vi "Insert Instrument Class by Name.vi"(8 "error in (no error)":errorcluster, 9 "Type":T1, 10 "Instrument in":refnum<class "Instrument.lvclass">, 11 "Control Experiment in":refnum<class "Control Experiment.lvclass">) -> (0 "error out":errorcluster, 1 "Found?":bool, 2 "Instrument out":refnum<class "Instrument.lvclass">, 3 "Control Experiment out":refnum<class "Control Experiment.lvclass">)   [LabVIEW 2019, in "Control Experiment.lvclass"]
uses:
  Control Experiment.lvclass
  Typedefs/Instrument Types--combo.ctl
  <userlib>/LevyLab/Instrument Framework/SMOs/Instrument/Instrument.lvclass
  Typedefs/Instruments--cluster.ctl
  <userlib>/LevyLab/Krohn Hite 7008/Instrument.KH7008.lvclass
  <userlib>/LevyLab/Lockin-Multichannel/Instrument.Lockin/Instrument.Lockin.lvclass
  <userlib>/LevyLab/Instrument Framework/Instrument Types/Cryostat/Instrument.Cryostat.lvclass
  <userlib>/LevyLab/Instrument Framework/Instrument Types/CBridge/Instrument.CBridge.lvclass
  <userlib>/LevyLab/Instrument Framework/Instrument Types/Delay Line/Instrument.DelayLine.lvclass
  <userlib>/LevyLab/Instrument Framework/Instrument Types/Strain/Instrument.Strain.lvclass
  <userlib>/LevyLab/Instrument Framework/Instrument Types/VNA/Instrument.VNA.lvclass
  <userlib>/LevyLab/Instrument Framework/Instrument Types/VSource/Instrument.VSource.lvclass
  Control Experiment.lvclass/Control Experiment.ctl
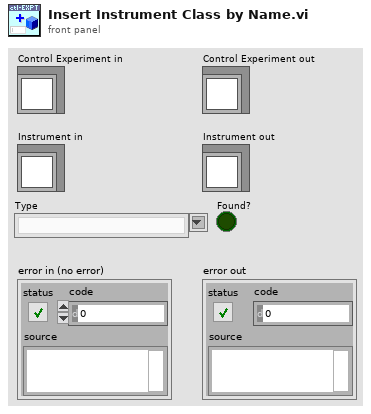
[diagram p1: front panel]
types:
  T1 = typedef "Control Experiment.lvclass/Instrument Types--combo.ctl" = string
  T2 = typedef "Control Experiment.lvclass/Instruments--cluster.ctl" = cluster{"KH7008":refnum<class "Instrument.KH7008.lvclass">[], "Lockin":refnum<class "Instrument.Lockin.lvclass">, "Temperature":refnum<class "Instrument.Cryostat.lvclass">, "Magnet":refnum<class "Instrument.Cryostat.lvclass">, "Rotator":refnum<class "Instrument.Cryostat.lvclass">, "Level":refnum<class "Instrument.Cryostat.lvclass">, "Capacitance Bridge":refnum<class "Instrument.CBridge.lvclass">, "Delay Line":refnum<class "Instrument.DelayLine.lvclass">, "Strain Cell":refnum<class "Instrument.Strain.lvclass">, "VNA":refnum<class "Instrument.VNA.lvclass">, "Voltage Source":refnum<class "Instrument.VSource.lvclass">}
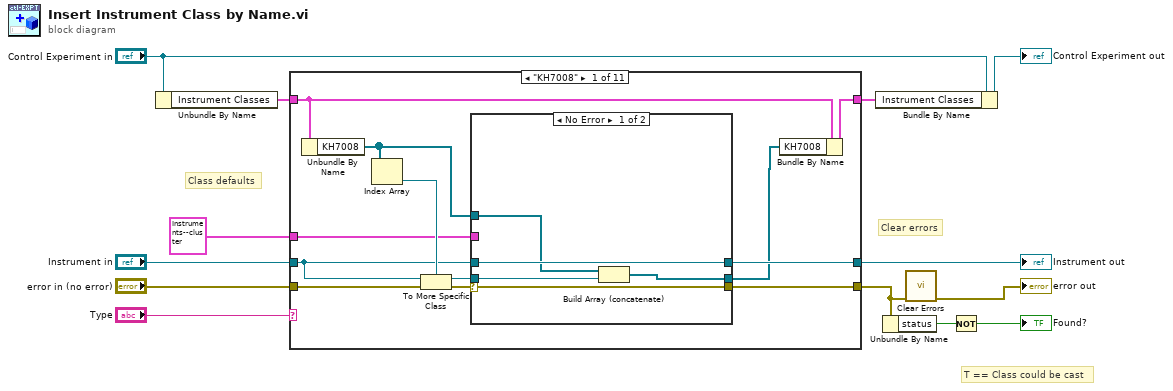
[diagram p0: block diagram]
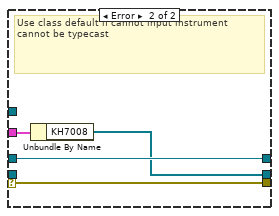
[diagram p2: hidden frame]
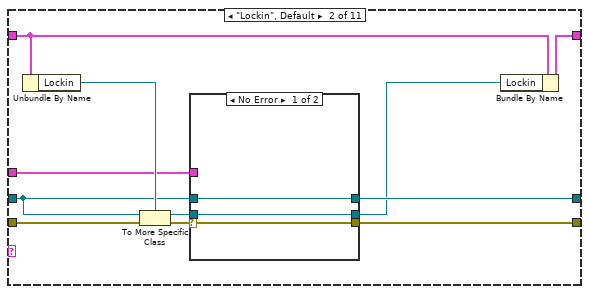
[diagram p3: hidden frame]
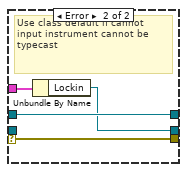
[diagram p4: hidden frame]
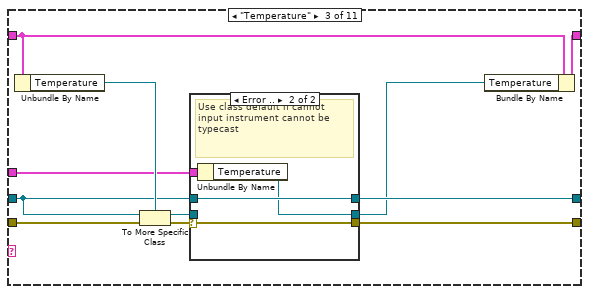
[diagram p5: hidden frame]
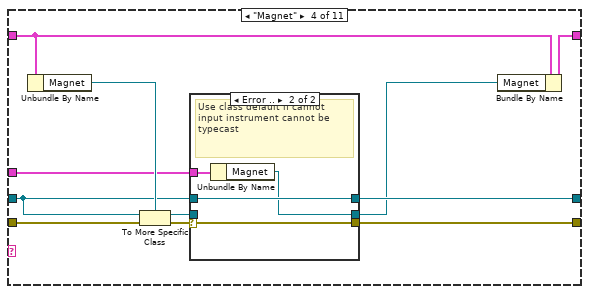
[diagram p7: hidden frame]
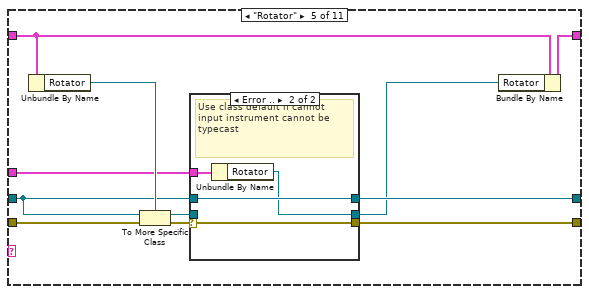
[diagram p9: hidden frame]
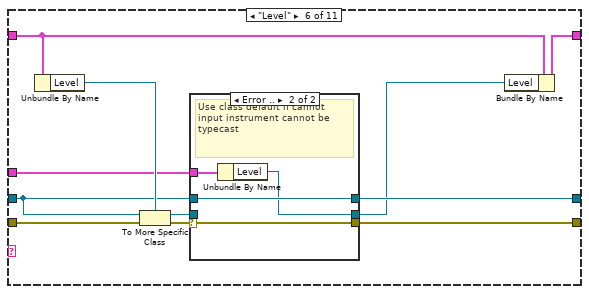
[diagram p11: hidden frame]
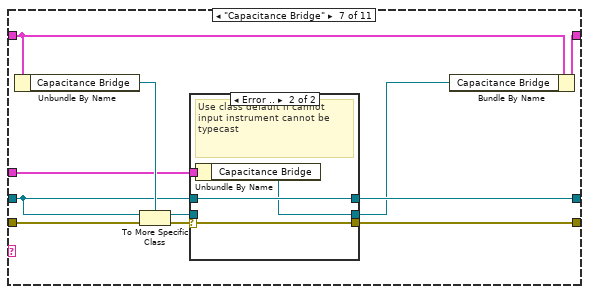
[diagram p13: hidden frame]
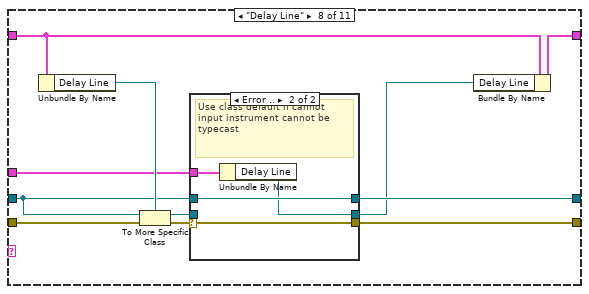
[diagram p15: hidden frame]
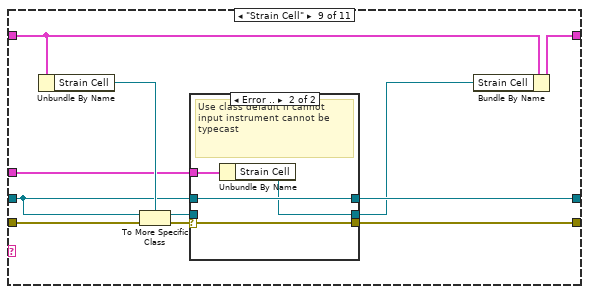
[diagram p17: hidden frame]
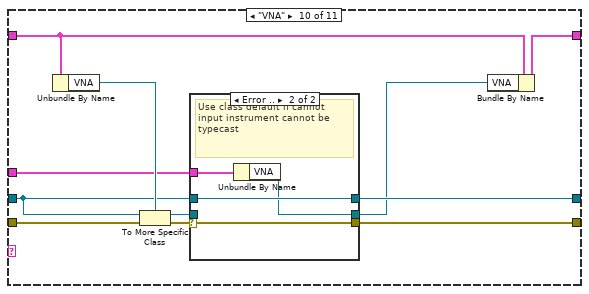
[diagram p19: hidden frame]
diagram:
  # "Class defaults"
  # "T == Class could be cast"
  # "Clear errors"
  n1 = Unbundle By Name("Control Experiment in") -> ("Instrument Classes"=w1:T2)
  n2 = case shown="\"KH7008\"" "Type" {
    tunnel: "Instrument in" -> [w17 w36 w54 w72 w90 w108 w126 w144 w162 w180 w198]
    tunnel: "error in (no error)" -> [w25 w45 w63 w81 w99 w117 w135 w153 w171 w189 w207]
    tunnel: [w16 w38 w56 w74 w92 w110 w128 w146 w164 w182 w200] -> w5
    tunnel: [w19 w39 w57 w75 w93 w111 w129 w147 w165 w183 w201] -> w10
    tunnel: [w23 w43 w61 w79 w97 w115 w133 w151 w169 w187 w205] -> w7
    tunnel: w1 -> [w24 w44 w62 w80 w98 w116 w134 w152 w170 w188 w206]
    tunnel: T2 {"KH7008"=[], "Lockin"=refnum, "Temperature"=refnum, "Magnet"=refnum, "Rotator"=refnum, "Level"=refnum, "Capacitance Bridge"=refnum, "Delay Line"=refnum, "Strain Cell"=refnum, "VNA"=refnum, "Voltage Source"=refnum} ("Instrument Classes") -> [w18 w37 w55 w73 w91 w109 w127 w145 w163 w181 w199]
    frame "KH7008" {
      n3 = Unbundle By Name(w24) -> ("KH7008"=w14:refnum<class "Instrument.KH7008.lvclass">[])
      n4 = Index Array(array=w14) -> (element=w22:refnum<class "Instrument.KH7008.lvclass">)  [unwired: 1 in]
      n5 = To More Specific Class(target class=w22, reference=w17, error in=w25) -> (specific class reference=w20:refnum<class "Instrument.KH7008.lvclass">, error out=w21:errorcluster)
      n6 = case shown="No Error" w21 {
        selector: w21 -> [w29 w33]
        tunnel: w20 -> [w28 _]
        tunnel: [w27 w31] -> w15
        tunnel: [w30 w34] -> w19
        tunnel: w17 -> [w30 w34]
        tunnel: [w29 w33] -> w16
        tunnel: w18 -> [_ w32]
        tunnel: w14 -> [w26 _]
        frame No Error {
          n7 = Build Array (concatenate)(w26, w28) -> (w27:refnum<class "Instrument.KH7008.lvclass">[])
        }
        frame Error {
          # "Use class default if cannot input instrument cannot be typecast"
          n8 = Unbundle By Name(w32) -> ("KH7008"=w31:refnum<class "Instrument.KH7008.lvclass">[])
        }
      }
      n9 = Bundle By Name(cluster=w24, "KH7008"=w15) -> (w23:T2)
    }
    frame "Lockin", Default {
      n10 = Unbundle By Name(w44) -> ("Lockin"=w42:refnum<class "Instrument.Lockin.lvclass">)
      n11 = To More Specific Class(target class=w42, reference=w36, error in=w45) -> (specific class reference=w40:refnum<class "Instrument.Lockin.lvclass">, error out=w41:errorcluster)
      n12 = case shown="No Error" w41 {
        selector: w41 -> [w46 w51]
        tunnel: w40 -> [w48 _]
        tunnel: [w48 w50] -> w35
        tunnel: [w47 w52] -> w39
        tunnel: w36 -> [w47 w52]
        tunnel: [w46 w51] -> w38
        tunnel: w37 -> [_ w49]
        frame No Error {
        }
        frame Error {
          # "Use class default if cannot input instrument cannot be typecast"
          n13 = Unbundle By Name(w49) -> ("Lockin"=w50:refnum<class "Instrument.Lockin.lvclass">)
        }
      }
      n14 = Bundle By Name(cluster=w44, "Lockin"=w35) -> (w43:T2)
    }
    frame "Temperature" {
      n15 = Unbundle By Name(w62) -> ("Temperature"=w60:refnum<class "Instrument.Cryostat.lvclass">)
      n16 = To More Specific Class(target class=w60, reference=w54, error in=w63) -> (specific class reference=w58:refnum<class "Instrument.Cryostat.lvclass">, error out=w59:errorcluster)
      n17 = case shown="Error .." w59 {
        selector: w59 -> [w64 w69]
        tunnel: w58 -> [w66 _]
        tunnel: [w66 w68] -> w53
        tunnel: [w65 w70] -> w57
        tunnel: w54 -> [w65 w70]
        tunnel: [w64 w69] -> w56
        tunnel: w55 -> [_ w67]
        frame No Error {
        }
        frame Error {
          # "Use class default if cannot input instrument cannot be typecast"
          n18 = Unbundle By Name(w67) -> ("Temperature"=w68:refnum<class "Instrument.Cryostat.lvclass">)
        }
      }
      n19 = Bundle By Name(cluster=w62, "Temperature"=w53) -> (w61:T2)
    }
    frame "Magnet" {
      n20 = Unbundle By Name(w80) -> ("Magnet"=w78:refnum<class "Instrument.Cryostat.lvclass">)
      n21 = To More Specific Class(target class=w78, reference=w72, error in=w81) -> (specific class reference=w76:refnum<class "Instrument.Cryostat.lvclass">, error out=w77:errorcluster)
      n22 = case shown="Error .." w77 {
        selector: w77 -> [w82 w87]
        tunnel: w76 -> [w84 _]
        tunnel: [w84 w86] -> w71
        tunnel: [w83 w88] -> w75
        tunnel: w72 -> [w83 w88]
        tunnel: [w82 w87] -> w74
        tunnel: w73 -> [_ w85]
        frame No Error {
        }
        frame Error {
          # "Use class default if cannot input instrument cannot be typecast"
          n23 = Unbundle By Name(w85) -> ("Magnet"=w86:refnum<class "Instrument.Cryostat.lvclass">)
        }
      }
      n24 = Bundle By Name(cluster=w80, "Magnet"=w71) -> (w79:T2)
    }
    frame "Rotator" {
      n25 = Unbundle By Name(w98) -> ("Rotator"=w96:refnum<class "Instrument.Cryostat.lvclass">)
      n26 = To More Specific Class(target class=w96, reference=w90, error in=w99) -> (specific class reference=w94:refnum<class "Instrument.Cryostat.lvclass">, error out=w95:errorcluster)
      n27 = case shown="Error .." w95 {
        selector: w95 -> [w100 w105]
        tunnel: w94 -> [w102 _]
        tunnel: [w102 w104] -> w89
        tunnel: [w101 w106] -> w93
        tunnel: w90 -> [w101 w106]
        tunnel: [w100 w105] -> w92
        tunnel: w91 -> [_ w103]
        frame No Error {
        }
        frame Error {
          # "Use class default if cannot input instrument cannot be typecast"
          n28 = Unbundle By Name(w103) -> ("Rotator"=w104:refnum<class "Instrument.Cryostat.lvclass">)
        }
      }
      n29 = Bundle By Name(cluster=w98, "Rotator"=w89) -> (w97:T2)
    }
    frame "Level" {
      n30 = Unbundle By Name(w116) -> ("Level"=w114:refnum<class "Instrument.Cryostat.lvclass">)
      n31 = To More Specific Class(target class=w114, reference=w108, error in=w117) -> (specific class reference=w112:refnum<class "Instrument.Cryostat.lvclass">, error out=w113:errorcluster)
      n32 = case shown="Error .." w113 {
        selector: w113 -> [w118 w123]
        tunnel: w112 -> [w120 _]
        tunnel: [w120 w122] -> w107
        tunnel: [w119 w124] -> w111
        tunnel: w108 -> [w119 w124]
        tunnel: [w118 w123] -> w110
        tunnel: w109 -> [_ w121]
        frame No Error {
        }
        frame Error {
          # "Use class default if cannot input instrument cannot be typecast"
          n33 = Unbundle By Name(w121) -> ("Level"=w122:refnum<class "Instrument.Cryostat.lvclass">)
        }
      }
      n34 = Bundle By Name(cluster=w116, "Level"=w107) -> (w115:T2)
    }
    frame "Capacitance Bridge" {
      n35 = Unbundle By Name(w134) -> ("Capacitance Bridge"=w132:refnum<class "Instrument.CBridge.lvclass">)
      n36 = To More Specific Class(target class=w132, reference=w126, error in=w135) -> (specific class reference=w130:refnum<class "Instrument.CBridge.lvclass">, error out=w131:errorcluster)
      n37 = case shown="Error .." w131 {
        selector: w131 -> [w136 w141]
        tunnel: w130 -> [w138 _]
        tunnel: [w138 w140] -> w125
        tunnel: [w137 w142] -> w129
        tunnel: w126 -> [w137 w142]
        tunnel: [w136 w141] -> w128
        tunnel: w127 -> [_ w139]
        frame No Error {
        }
        frame Error {
          # "Use class default if cannot input instrument cannot be typecast"
          n38 = Unbundle By Name(w139) -> ("Capacitance Bridge"=w140:refnum<class "Instrument.CBridge.lvclass">)
        }
      }
      n39 = Bundle By Name(cluster=w134, "Capacitance Bridge"=w125) -> (w133:T2)
    }
    frame "Delay Line" {
      n40 = Unbundle By Name(w152) -> ("Delay Line"=w150:refnum<class "Instrument.DelayLine.lvclass">)
      n41 = To More Specific Class(target class=w150, reference=w144, error in=w153) -> (specific class reference=w148:refnum<class "Instrument.DelayLine.lvclass">, error out=w149:errorcluster)
      n42 = case shown="Error .." w149 {
        selector: w149 -> [w154 w159]
        tunnel: w148 -> [w156 _]
        tunnel: [w156 w158] -> w143
        tunnel: [w155 w160] -> w147
        tunnel: w144 -> [w155 w160]
        tunnel: [w154 w159] -> w146
        tunnel: w145 -> [_ w157]
        frame No Error {
        }
        frame Error {
          # "Use class default if cannot input instrument cannot be typecast"
          n43 = Unbundle By Name(w157) -> ("Delay Line"=w158:refnum<class "Instrument.DelayLine.lvclass">)
        }
      }
      n44 = Bundle By Name(cluster=w152, "Delay Line"=w143) -> (w151:T2)
    }
    frame "Strain Cell" {
      n45 = Unbundle By Name(w170) -> ("Strain Cell"=w168:refnum<class "Instrument.Strain.lvclass">)
      n46 = To More Specific Class(target class=w168, reference=w162, error in=w171) -> (specific class reference=w166:refnum<class "Instrument.Strain.lvclass">, error out=w167:errorcluster)
      n47 = case shown="Error .." w167 {
        selector: w167 -> [w172 w177]
        tunnel: w166 -> [w174 _]
        tunnel: [w174 w176] -> w161
        tunnel: [w173 w178] -> w165
        tunnel: w162 -> [w173 w178]
        tunnel: [w172 w177] -> w164
        tunnel: w163 -> [_ w175]
        frame No Error {
        }
        frame Error {
          # "Use class default if cannot input instrument cannot be typecast"
          n48 = Unbundle By Name(w175) -> ("Strain Cell"=w176:refnum<class "Instrument.Strain.lvclass">)
        }
      }
      n49 = Bundle By Name(cluster=w170, "Strain Cell"=w161) -> (w169:T2)
    }
    frame "VNA" {
      n50 = Unbundle By Name(w188) -> ("VNA"=w186:refnum<class "Instrument.VNA.lvclass">)
      n51 = To More Specific Class(target class=w186, reference=w180, error in=w189) -> (specific class reference=w184:refnum<class "Instrument.VNA.lvclass">, error out=w185:errorcluster)
      n52 = case shown="Error .." w185 {
        selector: w185 -> [w190 w195]
        tunnel: w184 -> [w192 _]
        tunnel: [w192 w194] -> w179
        tunnel: [w191 w196] -> w183
        tunnel: w180 -> [w191 w196]
        tunnel: [w190 w195] -> w182
        tunnel: w181 -> [_ w193]
        frame No Error {
        }
        frame Error {
          # "Use class default if cannot input instrument cannot be typecast"
          n53 = Unbundle By Name(w193) -> ("VNA"=w194:refnum<class "Instrument.VNA.lvclass">)
        }
      }
      n54 = Bundle By Name(cluster=w188, "VNA"=w179) -> (w187:T2)
    }
    frame "Voltage Source" {
      n55 = Unbundle By Name(w206) -> ("Voltage Source"=w204:refnum<class "Instrument.VSource.lvclass">)
      n56 = To More Specific Class(target class=w204, reference=w198, error in=w207) -> (specific class reference=w202:refnum<class "Instrument.VSource.lvclass">, error out=w203:errorcluster)
      n57 = case shown="Error .." w203 {
        selector: w203 -> [w208 w213]
        tunnel: w202 -> [w210 _]
        tunnel: [w210 w212] -> w197
        tunnel: [w209 w214] -> w201
        tunnel: w198 -> [w209 w214]
        tunnel: [w208 w213] -> w200
        tunnel: w199 -> [_ w211]
        frame No Error {
        }
        frame Error {
          # "Use class default if cannot input instrument cannot be typecast"
          n58 = Unbundle By Name(w211) -> ("Voltage Source"=w212:refnum<class "Instrument.VSource.lvclass">)
        }
      }
      n59 = Bundle By Name(cluster=w206, "Voltage Source"=w197) -> (w205:T2)
    }
  }
  "Instrument out" <- w10
  n60 = Bundle By Name(cluster="Control Experiment in", "Instrument Classes"=w7) -> (→"Control Experiment out":refnum<class "Control Experiment.lvclass">)
  n61 = Unbundle By Name(w5) -> ("status"=w4:bool)
  n62 = call <vilib>:"Clear Errors.vi"("error in (no error)"=w5) -> ("error out"=→"error out":errorcluster)  [unwired: 5 in, 1 out]
  n63 = Not(x=w4) -> (.not. x?=→"Found?":bool)
